vi "getData_vX.vi"() -> ()   [LabVIEW 2014]
uses:
  <vilib>/FPGAPlugInAG/cRIO-9039/niLvFpga_Open_cRIO-9039.vi
  <vilib>/Utility/error.llb/Error Cluster From Error Code.vi
  <vilib>/rvi/errors/niLvFpgaAdjustHostInterfaceError.vi
  <vilib>/Utility/file.llb/Write To Spreadsheet File (DBL).vi
  <vilib>/FPGAPlugInAG/cRIO-9039/niLvFpga_Close_cRIO-9039.vi
  <vilib>/rvi/interface/nirviOpenFPGA/nirviOpenFPGA.xnode
  FPGA Bitfiles/test0304_FPGATarget_imptestv5_Y0EOgfHiaCk.lvbitx
  FPGA VIs/imp_test_v5.vi
  <vilib>/rvi/interface/nirviMethod/nirviMethod.xnode
  <vilib>/rvi/interface/nirviCloseFPGA/nirviCloseFPGA.xnode
  <vilib>/FPGAPlugInAG/cRIO-9039/niLvFpga_ReadFifo_cRIO-9039.vi
  <vilib>/rvi/errors/niLvFpgaMergeErrorWithErrorCode.vi
panel:
  in  "File path":path
  out "Timer (Sec)":u32
  out "FIFO empty":bool
  out "Elements Remaining":u32=10000
  in  "Time_read":i32=10000
  out "message":string=" INSTRUCTIONS:\r\rNormal Use:  When using subVIs that incorporate the error in/error out (or error I/O) structure, place this handler where you want to inform the user of an error, typically at the end of the I/O data path, as the last action of the program.  If the error in error? is ERROR, the handler creates a message describing the error and its source.  If the type of dialog = 1 (default), the message is displayed to the user, who can only acknowedge it.  If the type = 2, the user can acknowledge the message or abort execution; aborting a program with active I/O is not recommended.  If the type = 0, no message is displayed; this is used to process the error programmatically, and the error out cluster elements are wired to individual terminals for that reason.  \r\rOther Use:\n\r\nlocal testing.  To test the error code of a subVI or function that does not have the error I/O structure, you can wire its error code and a source string to the local error code and error source inputs.  If error in error? indicates no error and error code is not equal to 0, the local code and source are substituted for the error in values, and error? is set TRUE (ERROR)."
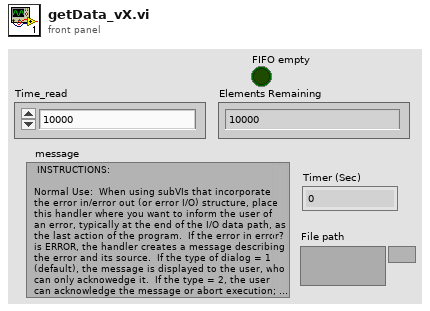
[diagram p1: front panel]
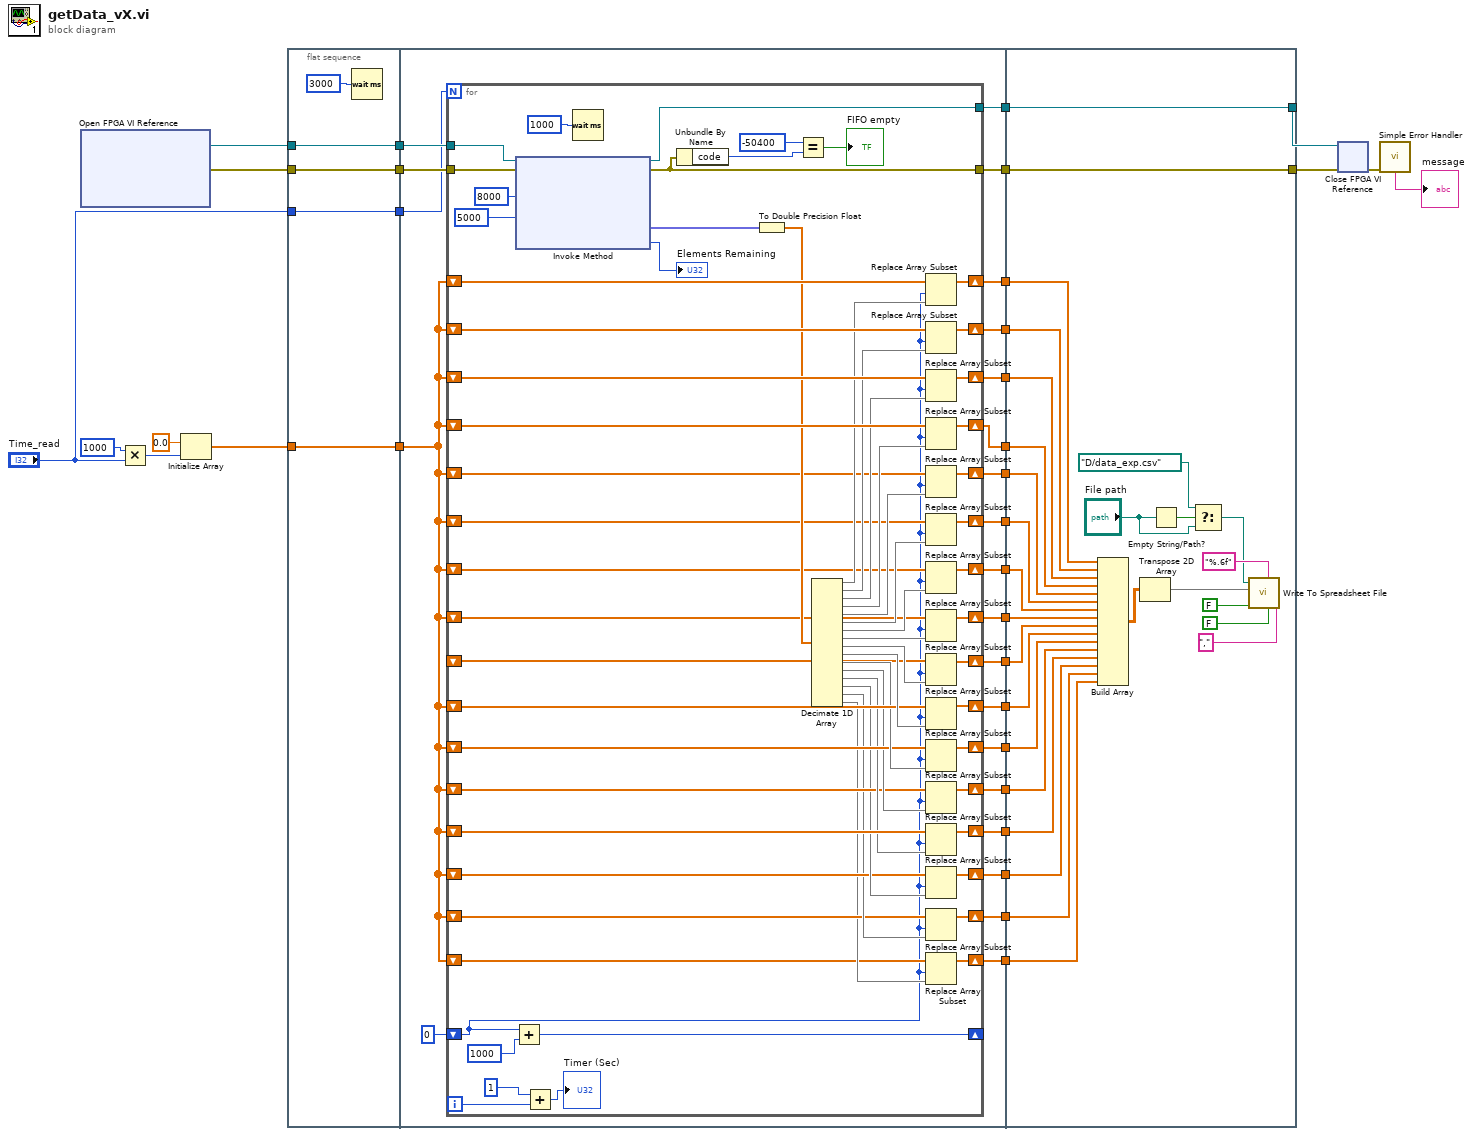
[diagram p0: block diagram]
diagram:
  n1 = xnode "Open FPGA VI Reference"() -> ("FPGA VI Reference Out"=w9:refnum<k20>, "error out"=w10:errorcluster)  [unwired: 2 in]
  n2 = Multiply(x=1000 ("y"), y="Time_read") -> (x*y=w26:i32)
  n3 = Initialize Array(0.0 ("element"), w26) -> (w30:dbl[])
  n4 = flat-sequence {
    tunnel: "Time_read" -> [w35]
    tunnel: w10 -> [w36]
    tunnel: w9 -> [w37]
    tunnel: w30 -> [w38]
    tunnel: [w38] -> w14
    tunnel: [w37] -> w13
    tunnel: [w36] -> w12
    tunnel: [w35] -> w11
    tunnel: [w58] -> w24
    tunnel: [w57] -> w23
    tunnel: [w56] -> w22
    tunnel: [w55] -> w21
    tunnel: [w54] -> w20
    tunnel: [w53] -> w19
    tunnel: [w52] -> w18
    tunnel: [w51] -> w17
    tunnel: [w50] -> w16
    tunnel: [w49] -> w15
    tunnel: w14 -> [w47]
    tunnel: w13 -> [w60]
    tunnel: w12 -> [w59]
    tunnel: w11 -> [w48]
    tunnel: [w46] -> w8
    tunnel: [w45] -> w7
    tunnel: [w44] -> w6
    tunnel: [w43] -> w5
    tunnel: [w42] -> w4
    tunnel: [w41] -> w3
    tunnel: [w40] -> w2
    tunnel: [w39] -> w1
    tunnel: w24 -> [w153]
    tunnel: w23 -> [w152]
    tunnel: w22 -> [w151]
    tunnel: [w156] -> w29
    tunnel: w21 -> [w156]
    tunnel: [w155] -> w28
    tunnel: w20 -> [w155]
    tunnel: w19 -> [w150]
    tunnel: w18 -> [w149]
    tunnel: w17 -> [w147]
    tunnel: w16 -> [w148]
    tunnel: w15 -> [w154]
    tunnel: w8 -> [w140]
    tunnel: w7 -> [w139]
    tunnel: w6 -> [w138]
    tunnel: w5 -> [w137]
    tunnel: w4 -> [w136]
    tunnel: w3 -> [w135]
    tunnel: w2 -> [w134]
    tunnel: w1 -> [w133]
    frame #0 {
      n5 = Wait (ms)(milliseconds to wait=u32 3000 ("y")) -> ()  [unwired: 1 out]
    }
    frame #1 {
      n6 = for {
        N: w48 -> [_]
        shift-right: [w126] -> _
        shift-left: 0 -> [w62]
        shift-right: [w115] -> w58
        shift-left: w47 -> [w124]
        shift-right: [w114] -> w57
        shift-left: w47 -> [w123]
        shift-right: [w113] -> w56
        shift-left: w47 -> [w122]
        shift-right: [w116] -> w49
        shift-left: w47 -> [w125]
        tunnel: w60 -> [w97]
        tunnel: w59 -> [w96]
        tunnel: [w92] -> w55
        tunnel: [w93] -> w54
        shift-right: [w107] -> w53
        shift-left: w47 -> [w108]
        shift-right: [w105] -> w52
        shift-left: w47 -> [w106]
        shift-right: [w104] -> w50
        shift-left: w47 -> [w103]
        shift-right: [w101] -> w51
        shift-left: w47 -> [w102]
        shift-right: [w85] -> w45
        shift-left: w47 -> [w84]
        shift-right: [w83] -> w44
        shift-left: w47 -> [w81]
        shift-right: [w80] -> w42
        shift-left: w47 -> [w79]
        shift-right: [w76] -> w43
        shift-left: w47 -> [w75]
        shift-right: [w73] -> w41
        shift-left: w47 -> [w72]
        shift-right: [w70] -> w40
        shift-left: w47 -> [w69]
        shift-right: [w67] -> w46
        shift-left: _ -> [w66]
        shift-right: [w64] -> w39
        shift-left: w47 -> [w63]
        i -> [w89]
        n7 = Add(x=w62, y=1000) -> (x+y=w126:i32)
        n8 = xnode "Invoke Method"("FPGA VI Reference In"=w97, "error in"=w96, "Number of Elements"=u32 8000, "Timeout (ms)"=5000) -> ("FPGA VI Reference Out"=w92:refnum<k20>, "error out"=w93:errorcluster, "Data"=w90:fxp<+/-,45,25>[], "Elements Remaining"=→"Elements Remaining":u32)
        n9 = Add(x=1, y=w89) -> (x+y=→"Timer (Sec)":i32)
        n10 = Wait (ms)(milliseconds to wait=u32 1000 ("y")) -> ()  [unwired: 1 out]
        n11 = Unbundle By Name(w93) -> ("code"=w99:i32)
        n12 = To Double Precision Float(number=w90) -> (double precision float=w121:dbl[])
        n13 = Equal?(x=-50400 ("y"), y=w99) -> (x = y?=→"FIFO empty":bool)
        n14 = Decimate 1D Array(w121) -> (w120:dbl[], w119:dbl[], w118:dbl[], w117:dbl[], w112:dbl[], w111:dbl[], w110:dbl[], w109:dbl[], w68:dbl[], w86:dbl[], w82:dbl[], w77:dbl[], w78:dbl[], w74:dbl[], w71:dbl[], w65:dbl[])
        n15 = Replace Array Subset(array=w125, new element=w120, index=w62) -> (w116:dbl[])
        n16 = Replace Array Subset(array=w124, new element=w119, index=w62) -> (w115:dbl[])
        n17 = Replace Array Subset(array=w123, new element=w118, index=w62) -> (w114:dbl[])
        n18 = Replace Array Subset(array=w122, new element=w117, index=w62) -> (w113:dbl[])
        n19 = Replace Array Subset(array=w108, new element=w112, index=w62) -> (w107:dbl[])
        n20 = Replace Array Subset(array=w106, new element=w111, index=w62) -> (w105:dbl[])
        n21 = Replace Array Subset(array=w103, new element=w110, index=w62) -> (w104:dbl[])
        n22 = Replace Array Subset(array=w102, new element=w109, index=w62) -> (w101:dbl[])
        n23 = Replace Array Subset(array=w66, new element=w68, index=w62) -> (w67:dbl[])
        n24 = Replace Array Subset(array=w84, new element=w86, index=w62) -> (w85:dbl[])
        n25 = Replace Array Subset(array=w81, new element=w82, index=w62) -> (w83:dbl[])
        n26 = Replace Array Subset(array=w75, new element=w77, index=w62) -> (w76:dbl[])
        n27 = Replace Array Subset(array=w79, new element=w78, index=w62) -> (w80:dbl[])
        n28 = Replace Array Subset(array=w72, new element=w74, index=w62) -> (w73:dbl[])
        n29 = Replace Array Subset(array=w69, new element=w71, index=w62) -> (w70:dbl[])
        n30 = Replace Array Subset(array=w63, new element=w65, index=w62) -> (w64:dbl[])
      }
    }
    frame #2 {
      n31 = Build Array(w154, w153, w152, w151, w150, w149, w148, w147, w140, w139, w138, w137, w136, w135, w134, w133) -> (w141:dbl[][])
      n32 = Transpose 2D Array(2D array=w141) -> (transposed array=w145:dbl[][])
      n33 = Empty String/Path?(string/path="File path") -> (empty?=w132:bool)
      n34 = Select(t=path "D:/data_exp.csv" ("file path (dialog if empty)"), s=w132, f="File path") -> (s? t:f=w129:path)
      n35 = call-poly <vilib>:"Write To Spreadsheet File.vi"("delimiter (\\t)"="," ("delimiter (\\t)"), "transpose? (no:F)"=FALSE, "format (%.3f)"="%.6f" ("format (%d)"), "append to file? (new file:F)"=FALSE, "2D data"=w145, "file path (dialog if empty)"=w129) -> ()  [unwired: 2 in, 1 out]
    }
  }
  n36 = xnode "Close FPGA VI Reference"("FPGA VI Reference In"=w29, "error in"=w28) -> ("error out"=w32:errorcluster)
  n37 = call <vilib>:"Simple Error Handler.vi"("error in (no error)"=w32) -> ("message"=→"message":string)  [unwired: 4 in, 4 out]
